vi "find_element_REF_by_key_chain.vi"(5 "ignore IDs":bool, 7 "id chain":string[](array[string]), 8 "error in (no error)":errorcluster, 10 "key chain":string[](array[string]), 11 "element ref":refnum<k20>) -> (0 "error out":errorcluster, 1 "found?":bool, 2 "subelement ref":refnum<k20>)   [LabVIEW 2010, in "XMLElement.lvclass"]
uses:
  XMLElement.lvclass
  Program Files/National Instruments/LabVIEW 2010/resource/objmgr/DOMUserDefRef.rc
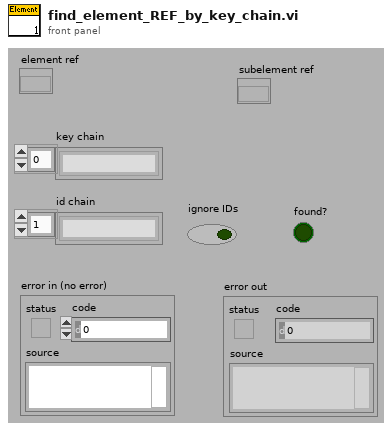
[diagram p1: front panel]
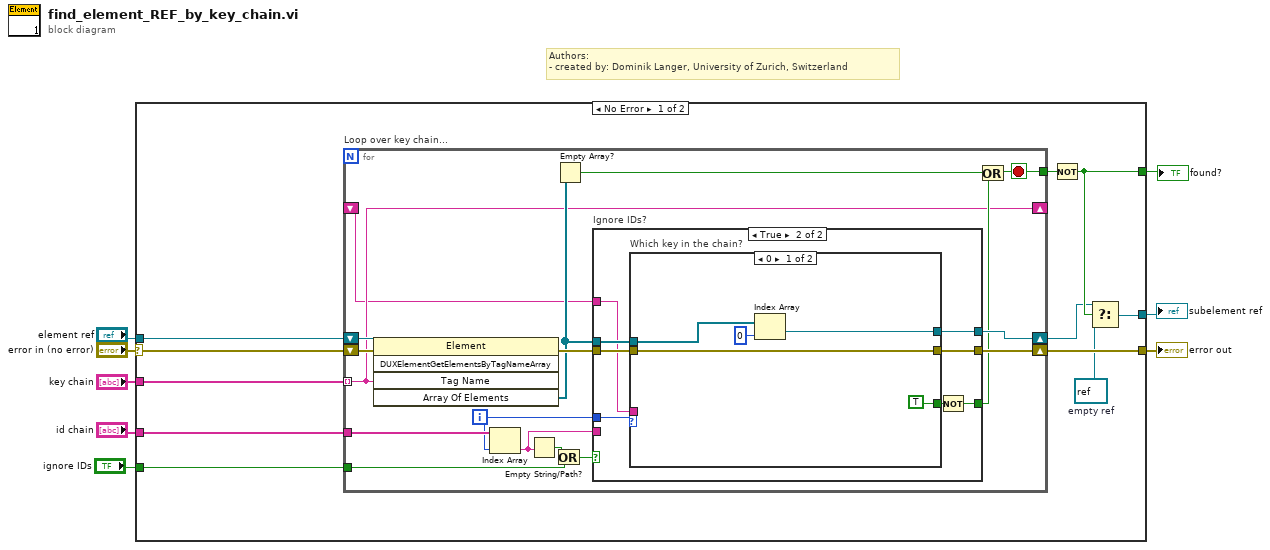
[diagram p0: block diagram]
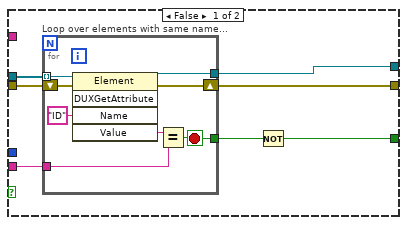
[diagram p2: hidden frame]
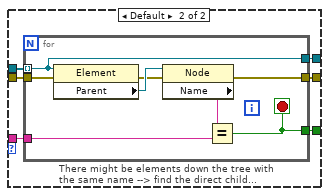
[diagram p3: hidden frame]
diagram:
  # "Authors: \n- created by: Dominik Langer, University of Zurich, Switzerland"
  n1 = case shown="No Error" "error in (no error)" {
    selector: "error in (no error)" -> [w9 w79]
    tunnel: [w17 w79] -> w7
    tunnel: "element ref" -> [w10 _]
    tunnel: "key chain" -> [w19 _]
    tunnel: "id chain" -> [w18 _]
    tunnel: [w12 _] -> w3
    tunnel: "ignore IDs" -> [w16 _]
    tunnel: [w14 _] -> w1
    frame No Error {
      w11 = refnum<k20> refnum  # empty ref
      n2 = for "Loop over key chain..." {
        shift-right: [w33] -> w17
        shift-left: w9 -> [w36]
        tunnel: w19 -> [w22] mode=indexing
        tunnel: w18 -> [w30]
        shift-right: [w34] -> w13
        shift-left: w10 -> [w35]
        tunnel: w16 -> [w28]
        tunnel: [w23] -> w15
        shift-right: [w22] -> _
        shift-left: _ -> [w21]
        i -> [w20]
        stop <- w23 stop-if-true
        n3 = invoke class="Element" method="DUXElementGetElementsByTagNameArray"(reference=w35, error in=w36, "Tag Name"=w22) -> (error out=w32:errorcluster, "Array Of Elements"=w31:refnum<k20>[])  [unwired: 2 in, 3 out]
        n4 = Index Array(array=w30, index=w20) -> (element=w26:string)
        n5 = Empty String/Path?(string/path=w26) -> (empty?=w29:bool)
        n6 = Or(x=w29, y=w28) -> (x .or. y?=w27:bool)
        n7 = Empty Array?(array=w31) -> (empty?=w24:bool)
        n8 = case "Ignore IDs?" shown="True" w27 {
          tunnel: [w43 w55] -> w34
          tunnel: [w42 w58] -> w33
          tunnel: w32 -> [w41 w59]
          tunnel: w31 -> [w40 w57]
          tunnel: w26 -> [w39 _]
          tunnel: [w37 w53] -> w25
          tunnel: w21 -> [_ w56]
          tunnel: w20 -> [_ w52]
          frame False {
            n9 = for "Loop over elements with same name..." {
              tunnel: w40 -> [w51] mode=indexing
              shift-right: [w49] -> w42
              shift-left: w41 -> [w50]
              tunnel: w39 -> [w47]
              tunnel: [w45] -> w43
              tunnel: [w44] -> w38
              stop <- w44 stop-if-true
              n10 = invoke class="Element" method="DUXGetAttribute"(reference=w51, error in=w50, "Name"="ID") -> (reference out=w45:refnum<k20>, error out=w49:errorcluster, "Value"=w46:string)  [unwired: 2 in, 2 out]
              n11 = Equal?(x=w46, y=w47) -> (x = y?=w44:bool)
            }
            n12 = Not(x=w38) -> (.not. x?=w37:bool)
          }
          frame True {
            n13 = case "Which key in the chain?" shown="0" w52 {
              tunnel: w59 -> [w62 w70]
              tunnel: [w62 w69] -> w58
              tunnel: w57 -> [w64 w68]
              tunnel: w56 -> [_ w67]
              tunnel: [w61 w66] -> w55
              tunnel: [TRUE w65] -> w54
              frame 0 {
                n14 = Index Array(array=w64, index=0) -> (element=w61:refnum<k20>)
              }
              frame Default {
                n15 = for "There might be elements down the tree with the same name --> find the direct child..." {
                  tunnel: w70 -> [w77]
                  tunnel: [w76] -> w69
                  tunnel: w68 -> [w72] mode=indexing
                  tunnel: w67 -> [w73]
                  tunnel: [w72] -> w66
                  tunnel: [w71] -> w65
                  stop <- w71 stop-if-true
                  n16 = property class="Element"(reference=w72, error in=w77) -> (error out=w75:errorcluster, "Parent"=w78:refnum<k20>)  [unwired: 1 out]
                  n17 = property class="Node"(reference=w78, error in=w75) -> (error out=w76:errorcluster, "Name"=w74:string)  [unwired: 1 out]
                  n18 = Equal?(x=w74, y=w73) -> (x = y?=w71:bool)
                }
              }
            }
            n19 = Not(x=w54) -> (.not. x?=w53:bool)
          }
        }
        n20 = Or(x=w24, y=w25) -> (x .or. y?=w23:bool)
      }
      n21 = Not(x=w15) -> (.not. x?=w14:bool)
      n22 = Select(t=w13, s=w14, f=w11) -> (s? t:f=w12:refnum<k20>)
    }
    frame Error {
    }
  }
  "error out" <- w7
  "subelement ref" <- w3
  "found?" <- w1
